vi "From Pythonic - String Array.vi"(4 "Pythonic Value":string) -> (1 "String Array":string[](array[string]))   [LabVIEW 2012, in "OPI.lvclass"]
doc: "Convert pythonic values into LabVIEW data. This method can be helpfull to convert elements of tuples or dictionaries.\n\nReturn a 1D array of string."
uses:
  OPI.lvclass
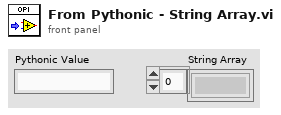
[diagram p1: front panel]
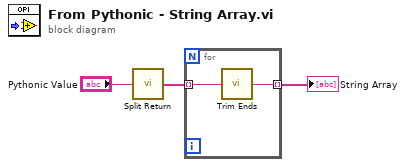
[diagram p0: block diagram]
diagram:
  n1 = call "Split Return.vi"("Return Value"="Pythonic Value") -> ("Split String"=w3:string[])
  n2 = for {
    tunnel: w3 -> [w5] mode=indexing
    tunnel: [w4] -> w2 mode=indexing
    n3 = call "Trim Ends.vi"("String"=w5) -> ("Trimmed String"=w4:string)
  }
  "String Array" <- w2
